vi "AOL Z Cal-Wizard.vi"   [LabVIEW 2017]
uses:
  Configuration code/Calibration/Globals/gl_Calibration globals.vi
types:
  T1 = typedef "FOV values cluster.ctl" = cluster{"Norm value":sgl, "FOV text":string, "FOV value":i32, "All FOV values":i32[], "All norm FOV values":sgl[], "All FOV value strings":string[], "Strings And Values []":T2}
  T2 = typedef "LVStringsAndValuesArrayTypeDef_SGL.ctl" = cluster{"String":string, "Value":sgl}[]
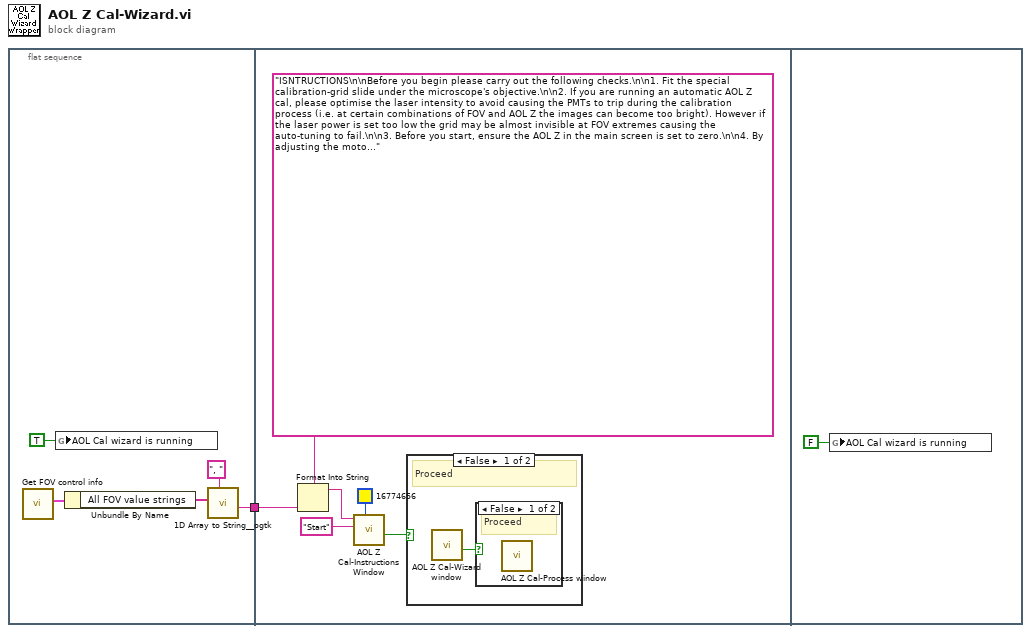
[diagram p0: block diagram]
diagram:
  n1 = flat-sequence {
    tunnel: [w2] -> w1
    tunnel: w1 -> [w8]
    frame #0 {
      n2 = call "Get FOV control info.vi"() -> ("FOV values cluster"=w3:T1)  [unwired: 8 in, 3 out]
      n3 = global write "gl_Calibration globals.vi" "AOL Cal wizard is running"(TRUE ("Motor Z Cal wizard is running")) -> ()
      n4 = Unbundle By Name(w3) -> ("All FOV value strings"=w4:string[])
      n5 = call <userlib>:"1D Array to String__ogtk.vi"("delimiter (Tab)"=", ", "Array of Strings"=w4) -> ("delimited string"=w2:string)  [unwired: 9 in]
    }
    frame #1 {
      n6 = Format Into String(format string="ISNTRUCTIONS\n\nBefore you begin please carry out the following checks.\n\n1. Fit the special calibration-grid slide under the microscope's objective.\n\n2. If you are running an automatic AOL Z cal, please optimise the laser intensity to avoid causing the PMTs to trip during the calibration process (i.e. at certain combinations of FOV and AOL Z the images can become too bright). However if the laser power is set too low the grid may be almost invisible at FOV extremes causing the auto-tuning to fail.\n\n3. Before you start, ensure the AOL Z in the main screen is set to zero.\n\n4. By adjusting the motor Z position focus perfectly on the calibration grid at the centre of the image (moving the stage downwards towards less positive Motor-Z values to minimise backlash error).\n\n5. Press the \"Set as Origin\" button in the main software screen to assign that Z position as the origin.\n\nThe motor will be calibrated for every field of view available (%s).\n\nStart the AOL Z calibration process?\n" ("Message string"), w8) -> (resulting string=w9:string)  [unwired: 2 in, 1 out]
      n7 = call "AOL Z Cal-Instructions Window.vi"("Colour"=u32 16774656, "Caption-Right button (OK)"="Start", "Message string"=w9) -> ("Cancelled (Left button pressed)"=w11:bool)  [unwired: 7 in, 1 out]
      n8 = case shown="False" w11 {
        frame False {
          # "Proceed"
          n9 = call "AOL Z Cal-Wizard window.vi"() -> ("Cancelled"=w13:bool)  [unwired: 10 in, 1 out]
          n10 = case shown="False" w13 {
            frame False {
              # "Proceed"
              n11 = call "AOL Z Cal-Process window.vi"() -> ()  [unwired: 9 in, 3 out]
            }
            frame True {
              # "Cancelled"
            }
          }
        }
        frame True {
          # "Cancelled"
        }
      }
    }
    frame #2 {
      n12 = global write "gl_Calibration globals.vi" "AOL Cal wizard is running"(FALSE ("Motor Z Cal wizard is running")) -> ()
    }
  }
